vi "Global Log.vi"() -> ()   [LabVIEW 2020, in "Logging.lvlib"]
uses:
  Logger Mananger/Logger Mananger.lvclass
  Logging.lvlib
panel:
  in  "Logger Mananger":refnum<class "Logger Mananger.lvclass">
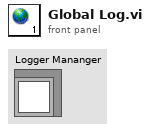
[diagram p1: front panel]
diagram:
